vi "IV Curve.vi"() -> ()   [LabVIEW 2016]
uses:
  <instrlib>/Keithley 24XX/Public/Data/Read (Single Point).vi
  <instrlib>/Keithley 24XX/Keithley 24XX.lvlib
panel:
  out "VR":cluster{dbl[], dbl[]}(graph)
  out "IR":cluster{dbl[], dbl[]}(graph)
  in  "2wire(F)/4wire(T)":bool=TRUE
  in  "Delay Time (s)":dbl=1.0
  in  "Output Base Directory":path=path "Z:/hsinyeh/LabViewToolBox/Data/IV_Curve"
  in  "moduleNumber":string="1"
  in  "fileName":string="test.txt"
  in  "Start":dbl
  in  "End Voltage ( V )":dbl=100.0
  in  "Interval ( V )":dbl=5.0
  in  "Source Mode  (0: Voltage)":u16(ring) items=["Voltage", "Current"]
  in  "Compliance  Level (0.1)":dbl=0.1
  in  "VISA resource name":refnum<visa-resource-name>="COM5"
  in  "Enable Resistance Auto Range (T:Enable)":bool=TRUE
  in  "Enable Current Auto Range (T:Enable)":bool=TRUE
  in  "Enable Voltage Auto Range (T:Enable)":bool=TRUE
  in  "Resistance Manual Range (1.0)":dbl=1.0
  in  "Current Manual Range (1.0)":dbl=1.0
  in  "Voltage Manual Range (1.0)":dbl=1.0
  in  "Serial Configuration":T1={"Baud Rate"=9600, "Parity"=0, "Data Bits"=8, "Stop Bits"=10, "Flow Control"=0} {"Flow Control" items=["None", "XON/XOFF", "RTS/CTS", "XON/XOFF & RTS/CTS", "DTR/DSR", "XON/XOFF & DTR/DSR"]; "Stop Bits" items=["1.0"=10, "1.5"=15, "2.0"=20]; "Data Bits" items=["7"=7, "8"=8]; "Parity" items=["None", "Odd", "Even", "Mark", "Space"]; "Baud Rate" items=["300"=300, "600"=600, "1200"=1200, "2400"=2400, "4800"=4800, "9600"=9600, "19200"=19200]}
  out "IV":cluster{dbl[], dbl[]}(graph)
  out "Resistance":sgl=-680628800000.0
  out "Current":sgl=-1.469503e-10
  out "Voltage":sgl=100.0186
  # "VR Curve"
  # "IR Curve"
  # "Settings"
  # "IV Curve with keithley 24XX source meter series\nHardware settings with RS-232\nMENU->COMMUNICATION->RS-232->Terminator-><LF>"
  # "Basic Settings (Don't need to change)"
  # "IV Curve"
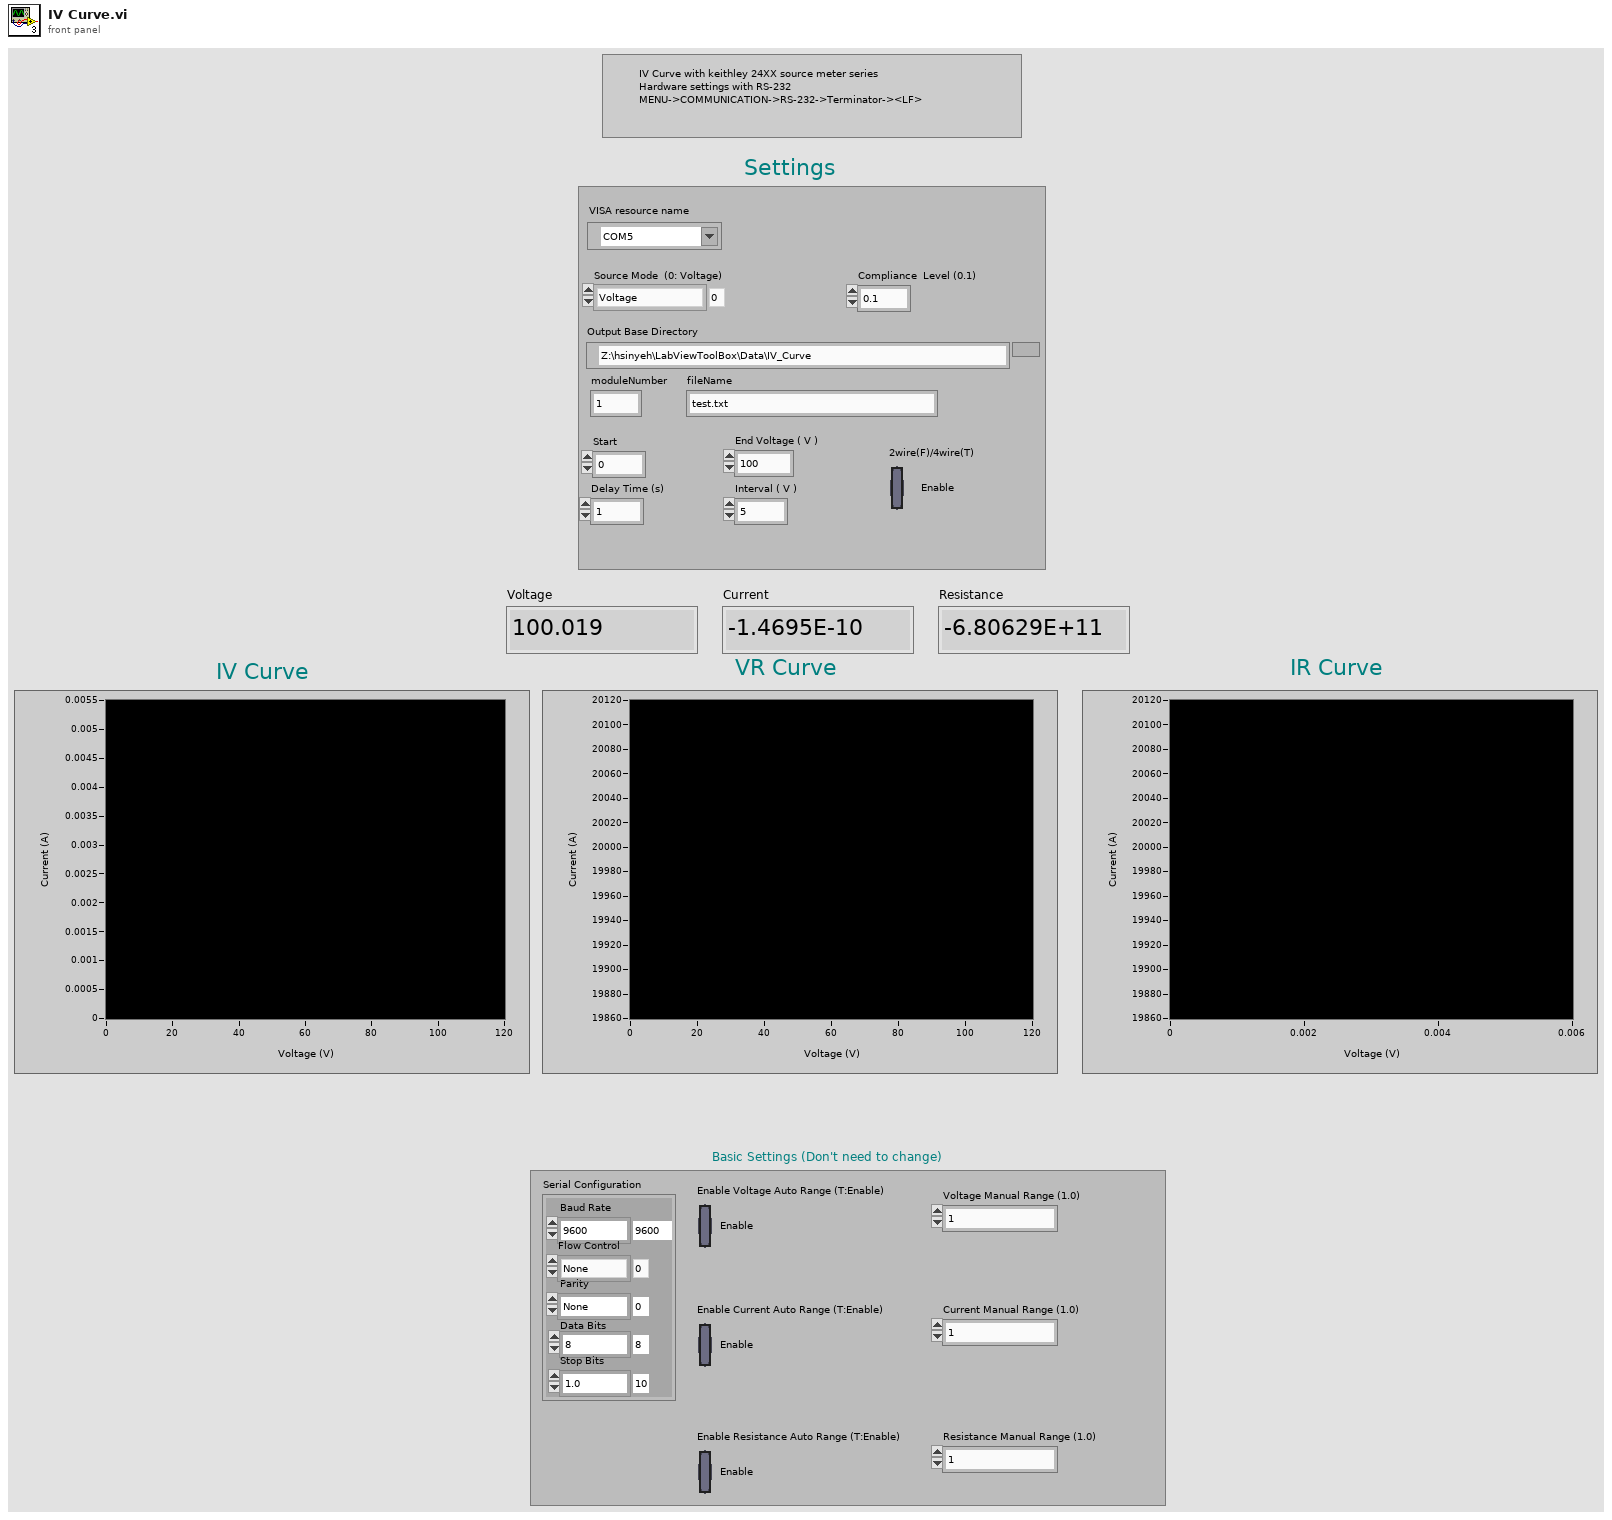
[diagram p1: front panel]
types:
  T1 = cluster{"Baud Rate":u32, "Parity":u16, "Data Bits":u16, "Stop Bits":u16, "Flow Control":u16}
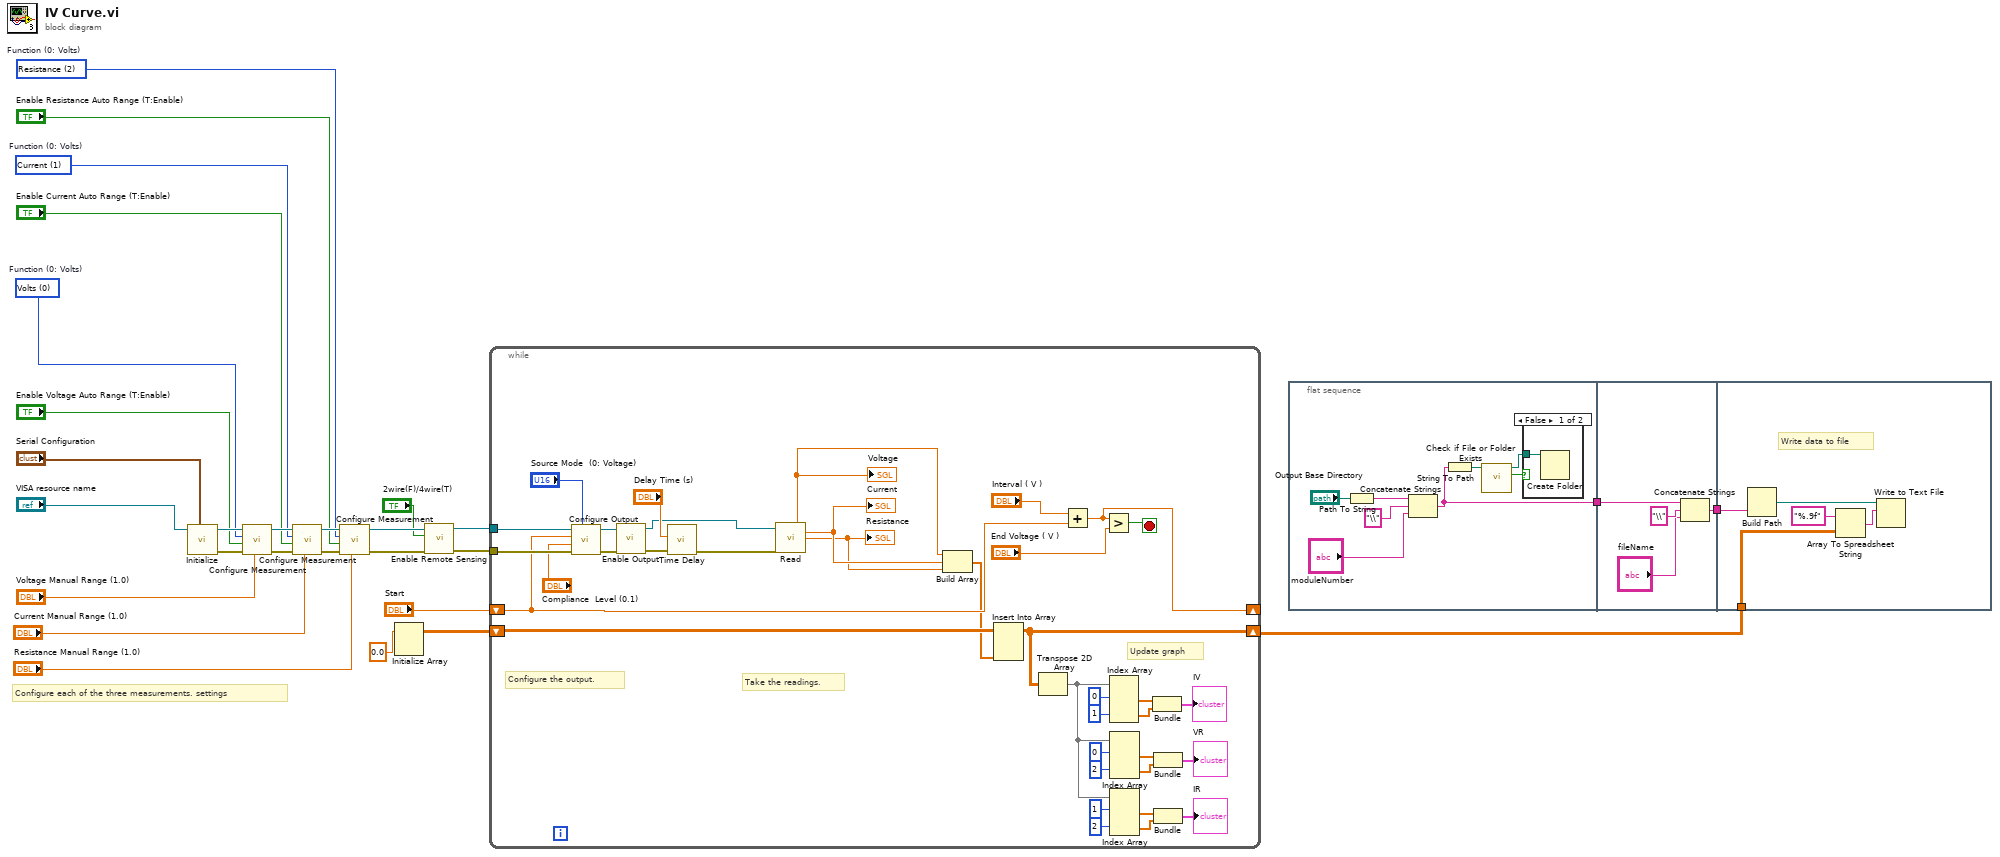
[diagram p0: block diagram]
diagram:
  w18 = u16 2 items=["Volts", "Current", "Resistance"]  # Function (0: Volts)
  w19 = u16 1 items=["Volts", "Current", "Resistance"]  # Function (0: Volts)
  w20 = u16 0 items=["Volts", "Current", "Resistance"]  # Function (0: Volts)
  # "Configure each of the three measurements. settings"
  n1 = call <instrlib>:"Initialize.vi"("Serial Configuration"="Serial Configuration", "VISA resource name"="VISA resource name") -> ("error out"=w25:errorcluster, "VISA resource name out"=w26:refnum<visa-resource-name>)  [unwired: 8 in]
  n2 = call <instrlib>:"Configure Measurement.vi"("Manual Range (1.0)"="Voltage Manual Range (1.0)", "error in (no error)"=w25, "Enable Auto Range (T:Enable)"="Enable Voltage Auto Range (T:Enable)", "Function (0: Volts)"=w20, "VISA resource name"=w26) -> ("error out"=w23:errorcluster, "VISA resource name out"=w24:refnum<visa-resource-name>)  [unwired: 5 in]
  n3 = call <instrlib>:"Configure Measurement.vi"("Manual Range (1.0)"="Current Manual Range (1.0)", "error in (no error)"=w23, "Enable Auto Range (T:Enable)"="Enable Current Auto Range (T:Enable)", "Function (0: Volts)"=w19, "VISA resource name"=w24) -> ("error out"=w22:errorcluster, "VISA resource name out"=w21:refnum<visa-resource-name>)  [unwired: 5 in]
  n4 = call <instrlib>:"Configure Measurement.vi"("Manual Range (1.0)"="Resistance Manual Range (1.0)", "error in (no error)"=w22, "Enable Auto Range (T:Enable)"="Enable Resistance Auto Range (T:Enable)", "Function (0: Volts)"=w18, "VISA resource name"=w21) -> ("error out"=w4:errorcluster, "VISA resource name out"=w5:refnum<visa-resource-name>)  [unwired: 5 in]
  n5 = Initialize Array(0.0 ("element")) -> (w6:dbl[][])  [unwired: 2 in]
  n6 = call <instrlib>:"Enable Remote Sensing.vi"("error in (no error)"=w4, "Enable Remote Sensing (T: Enable)"="2wire(F)/4wire(T)", "VISA resource name"=w5) -> ("error out"=w2:errorcluster, "VISA resource name out"=w3:refnum<visa-resource-name>)  [unwired: 7 in]
  n7 = while {
    tunnel: w2 -> [w64]
    tunnel: w3 -> [w65]
    shift-right: [w62] -> _
    shift-left: "Start" -> [w61]
    shift-right: [w57] -> w9
    shift-left: w6 -> [w63]
    stop <- w47 stop-if-true
    # "Configure the output."
    # "Update graph"
    # "Take the readings."
    n8 = call <instrlib>:"Configure Output.vi"("Source Mode  (0: Voltage)"="Source Mode  (0: Voltage)", "error in (no error)"=w64, "Compliance  Level (0.1)"="Compliance  Level (0.1)", "Output Level (0)"=w61, "VISA resource name"=w65) -> ("error out"=w43:errorcluster, "VISA resource name out"=w45:refnum<visa-resource-name>)  [unwired: 5 in]
    n9 = call <instrlib>:"Enable Output.vi"("error in (no error)"=w43, "VISA resource name"=w45) -> ("error out"=w42:errorcluster, "VISA resource name out"=w44:refnum<visa-resource-name>)  [unwired: 8 in]
    n10 = call "Time Delay"("error in (no error)"=w42, "Delay Time (s)"="Delay Time (s)") -> ("error out"=w49:errorcluster)  [unwired: 9 in]
    n11 = call-poly <instrlib>:"Read.vi"("VISA resource name"=w44, "error in (no error)"=w49) -> ("Voltage"=w52:sgl, "Current"=w53:sgl, "Resistance"=w46:sgl)  [unwired: 7 in, 4 out]
    "Voltage" <- w52
    "Current" <- w53
    "Resistance" <- w46
    n12 = Build Array(w52, w53, w46) -> (w54:sgl[])
    n13 = Insert Into Array(array=w63, new element=w54) -> (w57:dbl[][])  [unwired: 2 in]
    n14 = Transpose 2D Array(2D array=w57) -> (transposed array=w29:dbl[][])
    n15 = Add(x="Interval ( V )", y=w61) -> (x+y=w62:dbl)
    n16 = Greater?(x=w62, y="End Voltage ( V )") -> (0:w47:bool)
    n17 = Index Array(array=w29, index (row) #1=0 ("index (row)"), index (row) #2=1 ("index (row)")) -> (element #1=w59:dbl[], element #2=w60:dbl[])  [unwired: 2 in]
    n18 = Index Array(array=w29, index (row) #1=0 ("index (row)"), index (row) #2=2 ("index (row)")) -> (element #1=w38:dbl[], element #2=w39:dbl[])  [unwired: 2 in]
    n19 = Index Array(array=w29, index (row) #1=1 ("index (row)"), index (row) #2=2 ("index (row)")) -> (element #1=w33:dbl[], element #2=w34:dbl[])  [unwired: 2 in]
    n20 = Bundle(w59, w60) -> (→"IV":cluster{dbl[], dbl[]})  [unwired: 1 in]
    n21 = Bundle(w38, w39) -> (→"VR":cluster{dbl[], dbl[]})  [unwired: 1 in]
    n22 = Bundle(w33, w34) -> (→"IR":cluster{dbl[], dbl[]})  [unwired: 1 in]
  }
  n23 = flat-sequence {
    tunnel: [w73] -> w10
    tunnel: w10 -> [w78]
    tunnel: [w75] -> w8
    tunnel: w9 -> [w80]
    tunnel: w8 -> [w79]
    frame #0 {
      n24 = Path To String(path="Output Base Directory") -> (string=w68:string)
      n25 = Concatenate Strings(w68, "\\" ("string"), "moduleNumber") -> (w73:string)
      n26 = String To Path(string=w73) -> (path=w72:path)
      n27 = call <vilib>:"Check if File or Folder Exists.vi"("path"=w72) -> ("file or folder exists?"=w71:bool, "dup path"=w70:path)  [unwired: 8 in, 1 out]
      n28 = case shown="False" w71 {
        tunnel: w70 -> [w74 _]
        frame False {
          n29 = Create Folder(path (use dialog)=w74) -> ()  [unwired: 2 in, 3 out]
        }
        frame True {
        }
      }
    }
    frame #1 {
      n30 = Concatenate Strings(w78, "\\" ("string"), "fileName") -> (w75:string)
    }
    frame #2 {
      # "Write data to file"
      n31 = Build Path(name or relative path=w79) -> (appended path=w83:path)  [unwired: 1 in]
      n32 = Array To Spreadsheet String(array=w80, 3:"%.9f" ("format string")) -> (spreadsheet string=w82:string)  [unwired: 1 in]
      n33 = Write to Text File(file (use dialog)=w83, text=w82) -> ()  [unwired: 2 in, 3 out]
    }
  }
